vi "Toggle Channel.vi"(8 "error in":errorcluster, 9 "State":bool, 10 "Name":string, 11 "34980A in":refnum<class "34980A.lvclass">) -> (0 "error out":errorcluster, 3 "34980A out":refnum<class "34980A.lvclass">)   [LabVIEW 2019, in "34980A.lvlib" / "34980A.lvclass"]
uses:
  Library/34980A.lvclass
  C:/Users/Public/Documents/Development/builds/Instruments/MLTFNC.lvlibp/Library/MLTFNC.lvclass
  Library/34980A.lvclass/34980A.ctl
  builds/Instruments/MLTFNC.lvlibp/Accessors/Read Mapping.vi
  builds/Instruments/MLTFNC.lvlibp/Accessors/Read Channel_Index.vi
  builds/Instruments/MLTFNC.lvlibp/Library/MLTFNC.lvclass
  builds/Engine/Engine.lvlibp/Project/Engine.lvclass
  C:/Users/Public/Documents/Development/builds/Engine/Engine.lvlibp/Project/Engine.lvclass
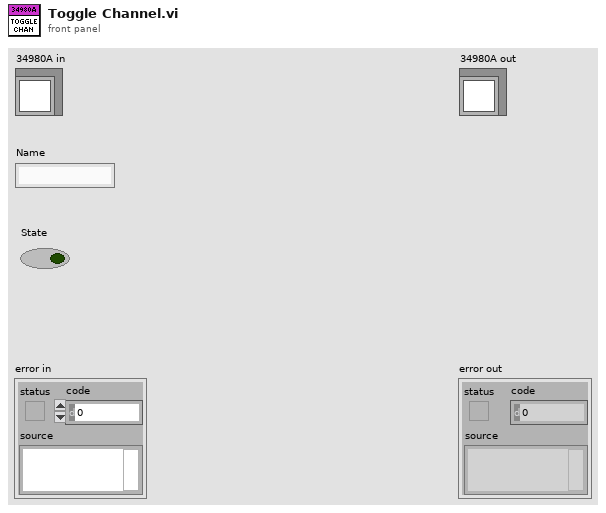
[diagram p1: front panel]
types:
  T1 = typedef "MLTFNC.lvlibp/MLTFNC.lvclass/Mapping.ctl" = cluster{"Address":u32[], "Bank":u32[], "Module":u32[], "Names":string[], "Routed":bool[]}
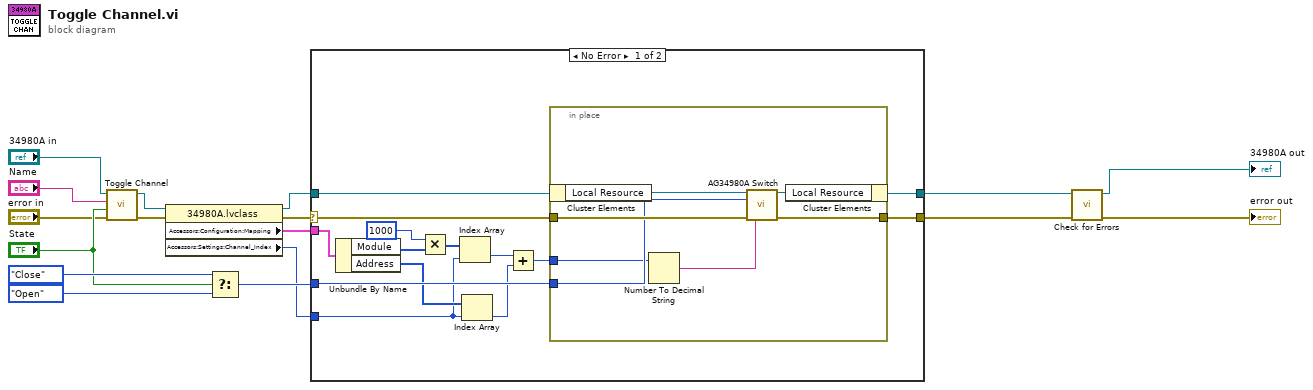
[diagram p0: block diagram]
diagram:
  n1 = call-parent "Toggle Channel.vi"("error in"="error in", "State"="State", "Name"="Name", "MLTFNC in"="34980A in") -> ("error out"=w9:errorcluster, "MLTFNC out"=w7:refnum<class "34980A.lvclass">)  [unwired: 6 in]
  n2 = property class="34980A.lvclass"(reference=w7, error in=w9) -> (reference out=w6:refnum<class "34980A.lvclass">, error out=w8:errorcluster, "Accessors:Configuration:Mapping"=w5:T1, "Accessors:Settings:Channel_Index"=w4:i32)
  n3 = Select(t=enum16{"Close", "Open"}."Close" ("Open/Close (0:Close)"), s="State", f=enum16{"Close", "Open"}."Open" ("Open/Close (0:Close)")) -> (s? t:f=w13:enum16{"Close", "Open"})
  n4 = case shown="No Error" w8 {
    selector: w8 -> [w27 w39]
    tunnel: w6 -> [w31 w40]
    tunnel: [w30 w40] -> w2
    tunnel: [w29 w39] -> w14
    tunnel: w13 -> [w28 _]
    tunnel: w5 -> [w26 _]
    tunnel: w4 -> [w19 _]
    frame No Error {
      n5 = Unbundle By Name(w26) -> ("Module"=w25:u32[], "Address"=w22:u32[])
      n6 = Multiply(x=1000, y=w25) -> (x*y=w23:u32[])
      n7 = Index Array(array=w23, index=w19) -> (element=w21:u32)
      n8 = Index Array(array=w22, index=w19) -> (element=w20:u32)
      n9 = Add(x=w21, y=w20) -> (x+y=w18:u32)
      n10 = in-place {
        in-place-border: w27 -> [w37]
        in-place-border: [w35] -> w29
        in-place-border: w28 -> [w33]
        in-place-border: w18 -> [w32]
        n11 = in-place-cluster #1(w31) -> ("Local Resource"=w38:refnum<visa-resource-name>)
        n12 = Number To Decimal String(number=w32) -> (decimal integer string=w34:string)  [unwired: 1 in]
        n13 = call <instrlib>:"AG34980A Switch.vi"("VISA resource name"=w38, "Channel List"=w34, "Open/Close (0:Close)"=w33, "error in (no error)"=w37) -> ("VISA resource name out"=w36:refnum<visa-resource-name>, "error out"=w35:errorcluster)  [unwired: 9 in, 1 out]
        n14 = in-place-cluster #1("Local Resource"=w36) -> (w30:refnum<class "34980A.lvclass">)
      }
    }
    frame Error {
    }
  }
  n15 = call "Check for Errors.vi"("error in"=w14, "Engine in"=w2) -> ("error out"=→"error out":errorcluster, "Engine out"=→"34980A out":refnum<class "34980A.lvclass">)  [unwired: 8 in]
